vi "Convert Tree Tag to VI and UID.vi"(11 "Tree Tag":string) -> (1 "Item Name":string, 2 "GObject UID":string, 3 "File Path (Relative)":string, 5 "UID Type":T1)   [LabVIEW 2013, in "SET Project Editor.lvlib"]
doc: "Convert Tree Tag to VI and UID.vi\n\nBreaks the unique item string into its components and identifies its type."
uses:
  SET Project Editor.lvlib
  Types/UID Types.ctl
panel:
  # "[VI Name]::[GObject UID].[Item Name]"
  # "[RTM Name]::[Item Name]"
  # "VI Name::GObject UID"
  # "Convert Tree Tag to VI and UID.vi\n\nBreaks the unique item string into its components and identifies its type."
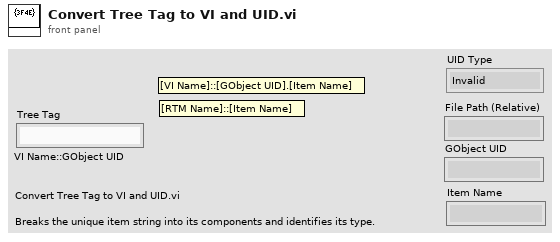
[diagram p1: front panel]
types:
  T1 = typedef "SET Project Editor.lvlib/UID Types.ctl" = enum16{"Invalid", "VI File", "GObject", "GObject Item", "RTM File", "RTM Item"}
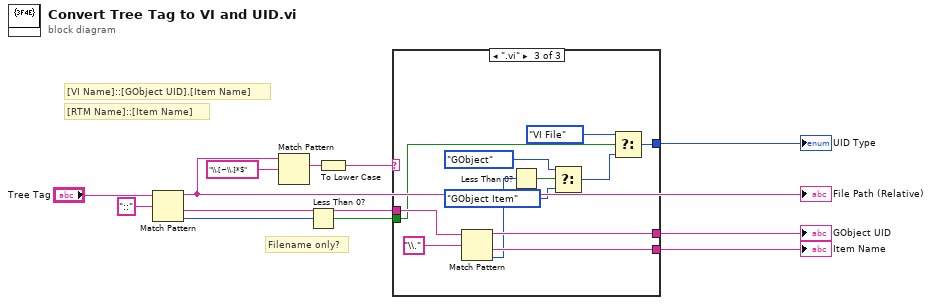
[diagram p0: block diagram]
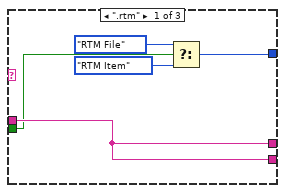
[diagram p2: hidden frame]
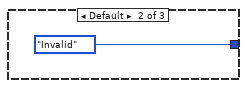
[diagram p3: hidden frame]
diagram:
  # "Filename only?"
  # "[RTM Name]::[Item Name]"
  # "[VI Name]::[GObject UID].[Item Name]"
  n1 = Match Pattern(string="Tree Tag", regular expression="::" ("search string/char (-)")) -> (before substring=w4:string, after substring=w9:string, offset past match=w7:i32)  [unwired: 1 in, 1 out]
  "File Path (Relative)" <- w4
  n2 = Match Pattern(string=w4, regular expression="\\.[~\\.]*$") -> (match substring=w5:string)  [unwired: 4 out]
  n3 = Less Than 0?(x=w7) -> (x < 0?=w2:bool)
  n4 = To Lower Case(string=w5) -> (all lower case string=w3:string)
  n5 = case shown="\".vi\"" w3 {
    tunnel: [w17 _ w30] -> w10
    tunnel: w9 -> [w17 _ w29]
    tunnel: [w17 _ w28] -> w8
    tunnel: w2 -> [w16 _ w26]
    tunnel: [w13 UID_Types."Invalid" w19] -> w1
    frame ".rtm" {
      n6 = Select(t=UID_Types."RTM File", s=w16, f=UID_Types."RTM Item") -> (s? t:f=w13:T1)
    }
    frame Default {
    }
    frame ".vi" {
      n7 = Match Pattern(string=w29, regular expression="\\.") -> (before substring=w28:string, after substring=w30:string, offset past match=w24:i32)  [unwired: 1 in, 1 out]
      n8 = Less Than 0?(x=w24) -> (x < 0?=w23:bool)
      n9 = Select(t=UID_Types."GObject", s=w23, f=UID_Types."GObject Item") -> (s? t:f=w20:T1)
      n10 = Select(t=UID_Types."VI File", s=w26, f=w20) -> (s? t:f=w19:T1)
    }
  }
  "GObject UID" <- w8
  "UID Type" <- w1
  "Item Name" <- w10
